vi "Get Step Size Burst Count.vi"(8 "error in (no error)":errorcluster, 11 "VISA resource name":refnum<visa-resource-name>) -> (0 "error out":errorcluster, 2 "Step Size Burst Count":i32, 3 "VISA resource name out":refnum<visa-resource-name>, 4 "Device Errors":cluster{"code":i32, "Text":string}[](array[cluster]))   [LabVIEW 2014, in "Stanford Research DG645 - Driver.lvlib"]
doc: "Burst Command: SSBZ?\nInstrument Error Check\n\nQuery current step size for the burst count."
uses:
  Stanford Research DG645 - Driver.lvlib
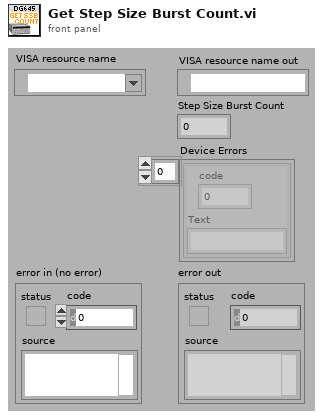
[diagram p1: front panel]
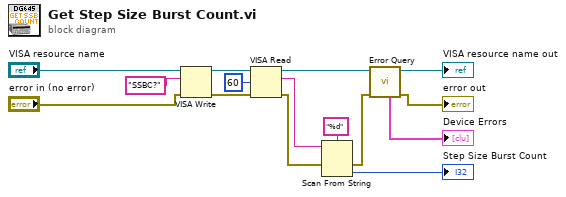
[diagram p0: block diagram]
diagram:
  n1 = VISA Write(VISA resource name="VISA resource name", write buffer="SSBC?" ("command"), error in (no error)="error in (no error)") -> (VISA resource name out=w14:refnum<visa-resource-name>, error out=w13:errorcluster)  [unwired: 1 out]
  n2 = VISA Read(VISA resource name=w14, byte count=u32 60, error in (no error)=w13) -> (VISA resource name out=w12:refnum<visa-resource-name>, read buffer=w9:string, error out=w5:errorcluster)  [unwired: 1 out]
  n3 = Scan From String(format string="%d", input string=w9, error in=w5) -> (error out=w4:errorcluster, output 1=→"Step Size Burst Count":i32)  [unwired: 2 in, 2 out]
  n4 = call "Error Query.vi"("error in (no error)"=w4, "VISA resource name"=w12) -> ("error out"=→"error out":errorcluster, "VISA resource name out"=→"VISA resource name out":refnum<visa-resource-name>, "Device Errors"=→"Device Errors":cluster{"code":i32, "Text":string}[])  [unwired: 7 in]
